vi "Read Teller.vi"(11 "Stopped Msg Input in":refnum<class "Stopped Msg Input.lvclass">) -> (2 "Teller":refnum<class "Teller.lvclass">)   [LabVIEW 2020, in "jettl.lvlib" / "Stopped jettl Msg.lvlib" / "Stopped Msg Input.lvlib" / "Stopped Msg Input.lvclass"]
uses:
  Stopped Msg Input.lvclass
  Teller/Teller.lvclass
  Stopped Msg Input.lvclass/Stopped Msg Input.ctl
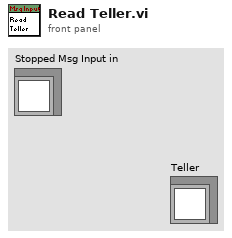
[diagram p1: front panel]
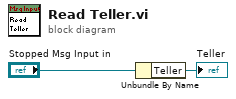
[diagram p0: block diagram]
diagram:
  n1 = Unbundle By Name("Stopped Msg Input in") -> ("Teller"=→"Teller":refnum<class "Teller.lvclass">)
